vi "Day 14 Task 2 attempt 3.vi"() -> ()   [LabVIEW 2018]
uses:
  <userlib>/_OpenG.lib/array/array.llb/Remove Duplicates from 1D Array (String)__ogtk.vi
  <userlib>/_OpenG.lib/array/array.llb/Sort 1D Array (String)__ogtk.vi
  <userlib>/_OpenG.lib/array/array.llb/Reorder 2D Array2 (U64)__ogtk.vi
panel:
  out "ANSWER":u64
  out "Letter combo":string[](array[string])
  out "Letter combos it turns into":string[](array[string])
  out "Array 9":string[](array[string])
  out "Array 8":string[](array[string])
  out "Array 7":string[][](array[string])
  out "sum":u64
  out "Array 6":u64[][](array[numeric])
  out "String":string
  out "how many of each":u64[](array[numeric])
  out "step":i32
  out "Numeric":i32
  out "Array 5":u64[][](array[numeric])
  out "no. pairs":u64[](graph)
  out "Masks for 2 letter combos":i16[][](array[numeric])
  out "Array":i64[](array[numeric])
  out "2 letter combos":string[](array[string])
  out "Letters used (single)":string[](array[string])
  out "Array 4":u64[](array[numeric])
  out "Array 3":u64[](array[numeric])
  out "Polymer template":string
  out "array":string[][](array[string])
  # "3 letters = 2 pairs\nno. letters = no. pairs + 1"
  # "1749+298+161+865=3073"
  # "7 letters = 6 pairs"
  # "CB"
  # "Template:     NNCB\nAfter step 1: NCNBCHB\nAfter step 2: NBCCNBBBCBHCB\nAfter step 3: NBBBCNCCNBBNBNBBCHBHHBCHB\nAfter step 4: NBBNBNBBCCNBCNCCNBBNBBNBBBNBBNBBCBHCBHHNHCBBCBHCB"
  # "BB= BN + HB"
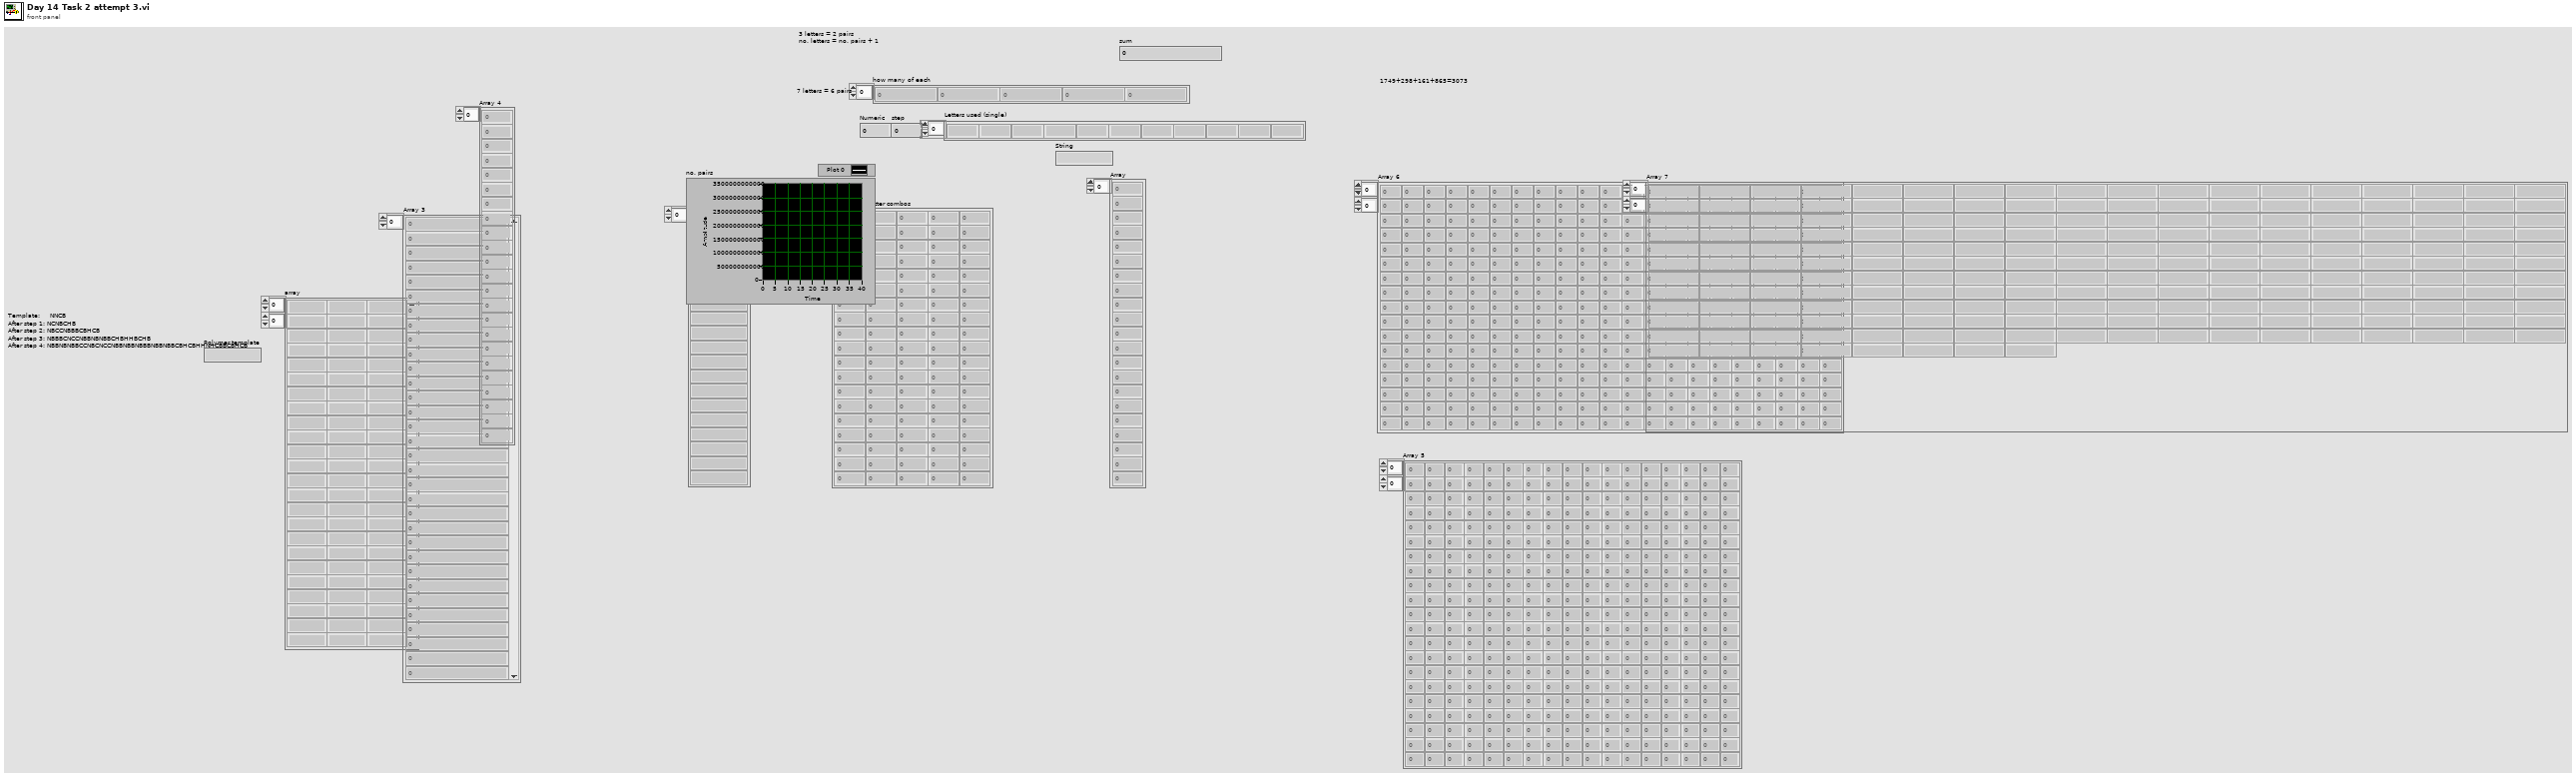
[diagram p1: front panel]
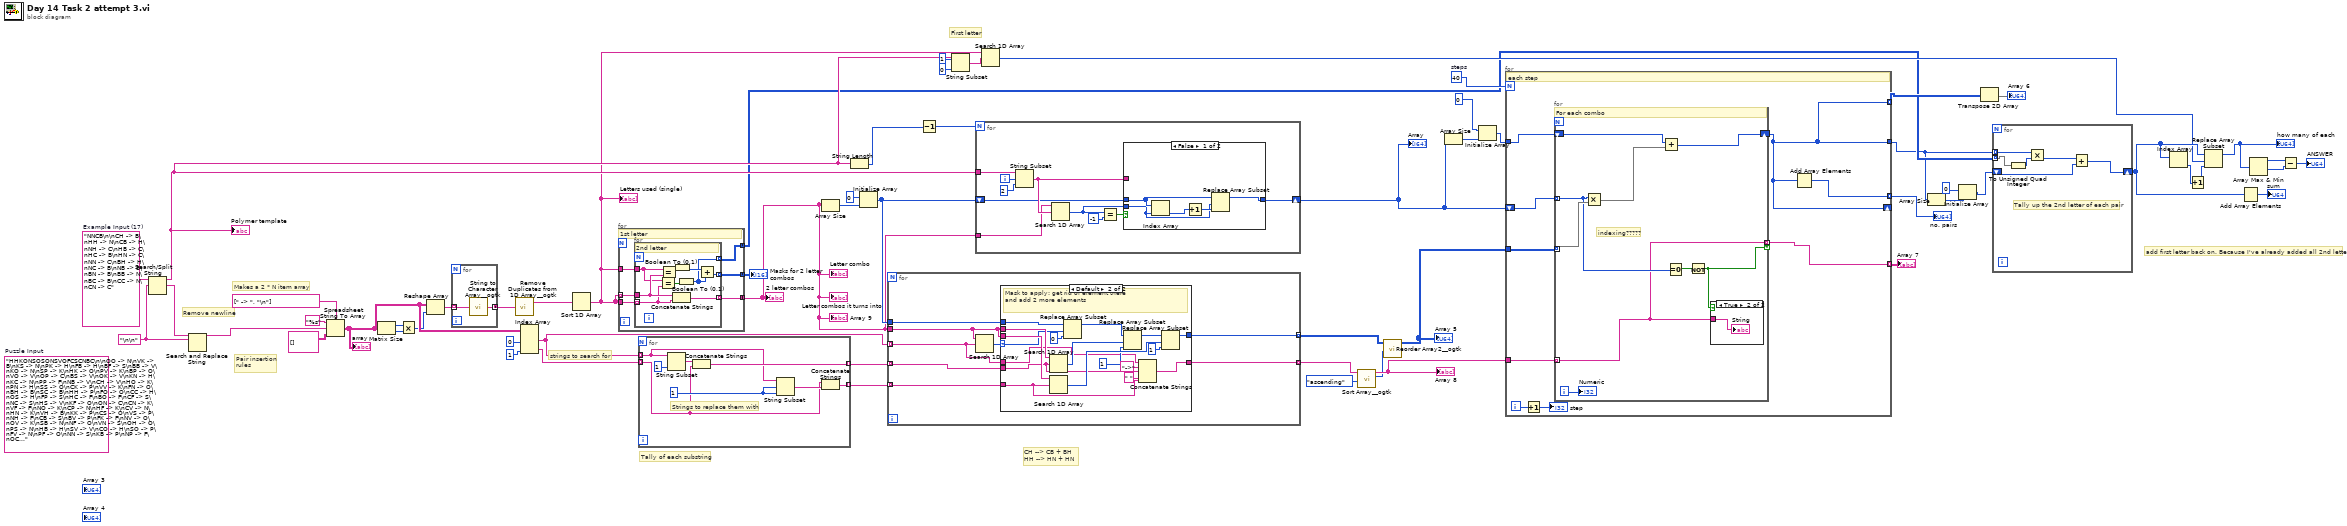
[diagram p0: block diagram]
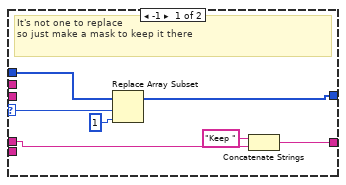
[diagram p3: hidden frame]
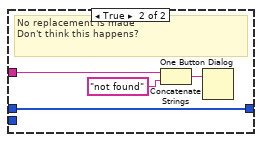
[diagram p4: hidden frame]
diagram:
  w38 = 40  # steps
  w57 = "\n\n" ("delimiter (Tab)")
  (unwired) "HHKONSOSONSVOFCSCNBC\n\nOO -> N\nVK -> B\nKS -> N\nPK -> H\nFB -> H\nBF -> S\nBB -> V\nKO -> N\nSP -> K\nHK -> O\nPV -> K\nBP -> O\nVO -> V\nOP -> C\nBS -> V\nOK -> V\nKN -> H\nKC -> N\nPP -> F\nNB -> V\nCH -> V\nHO -> K\nPN -> H\nSS -> O\nCK -> P\nVV -> K\nFN -> O\nBH -> B\nSC -> B\nHH -> P\nFO -> O\nCC -> H\nOS -> H\nFP -> S\nHC -> F\nBO -> F\nCF -> S\nNC -> S\nHS -> V\nKF -> O\nON -> C\nCN -> K\nVF -> F\nNO -> K\nCP -> N\nHF -> K\nCV -> N\nHN -> K\nVH -> B\nKK -> P\nCS -> O\nVS -> P\nNH -> F\nCB -> S\nBV -> P\nFK -> F\nNV -> O\nOV -> K\nSB -> N\nNF -> O\nVN -> S\nOH -> O\nPS -> N\nHB -> H\nSV -> V\nCO -> H\nSO -> P\nFV -> N\nPF -> O\nNN -> S\nKB -> P\nNP -> F\nOC -> S\nFS -> P\nFH -> P\nVP -> K\nBN -> O\nNS -> H\nVB -> V\nPO -> K\nKP -> N\nSN -> O\nBC -> H\nSF -> V\nPC -> O\nNK -> F\nBK -> V\nKH -> S\nSH -> S\nSK -> H\nOB -> V\nPH -> N\nPB -> C\nHV -> N\nHP -> V\nFF -> B\nOF -> P\nVC -> S\nKV -> C\nFC -> F"  # Puzzle Input
  w1 = "NNCB\n\nCH -> B\nHH -> N\nCB -> H\nNH -> C\nHB -> C\nHC -> B\nHN -> C\nNN -> C\nBH -> H\nNC -> B\nNB -> B\nBN -> B\nBB -> N\nBC -> B\nCC -> N\nCN -> C"  # Example Input (17)
  # "First letter"
  # "add first letter back on. Because I've already added all 2nd letters"
  # "strings to search for"
  # "CH --> CB + BH\nHH --> HN + HN"
  # "Pair insertion\nrules"
  # "Tally of each substring"
  # "Remove newline"
  # "Makes a 2 * N item array"
  n1 = Search/Split String(string=w1, search string/char (-)=w57) -> (substring before match=w18:string, match + rest of string=w58:string)  [unwired: 1 in, 1 out]
  "Polymer template" <- w18
  n2 = Search and Replace String(input string=w58, search string=w57) -> (result string=w56:string)  [unwired: 6 in, 3 out]
  n3 = Spreadsheet String To Array(delimiter (Tab)=string[] [" -> ", "\n"], format string="%s", spreadsheet string=w56, array type (2D Dbl)=string[][] []) -> (array=w55:string[][])
  "array" <- w55
  n4 = Matrix Size(0:w55) -> (1:w50:i32, 2:w51:i32)
  n5 = Multiply(x=w50, y=w51) -> (x*y=w49:i32)
  n6 = Reshape Array(w55, w49) -> (w47:string[])
  n7 = for {
    tunnel: w47 -> [w63] mode=indexing
    tunnel: [w62] -> w46 mode=concatenating
    n8 = call <userlib>:"String to Character Array__ogtk.vi"("Input String"=w63) -> ("Character Array"=w62:string[])
  }
  n9 = call-poly <userlib>:"Remove Duplicates from 1D Array__ogtk.vi"("Input Array"=w46) -> ("Output Array"=w27:string[])  [unwired: 1 out]
  n10 = Index Array(array=w55, index (col) #1=0 ("disabled index (col)"), index (col) #2=1 ("index (col)")) -> (element #1=w45:string[], element #2=w52:string[])  [unwired: 2 in]
  n11 = Sort 1D Array(array=w27) -> (sorted array=w15:string[])
  "Letters used (single)" <- w15
  n12 = for {
    tunnel: w15 -> [w68]
    tunnel: w15 -> [w69] mode=indexing
    tunnel: [w67] -> w39 mode=concatenating
    tunnel: w15 -> [w66]
    tunnel: [w65] -> w30 mode=concatenating
    tunnel: [w64] -> w5 mode=concatenating
    # "1st letter"
    n13 = for {
      tunnel: w69 -> [w77]
      tunnel: w68 -> [w76] mode=indexing
      tunnel: [w78] -> w67 mode=indexing
      tunnel: w66 -> [w75]
      tunnel: [w72] -> w65 mode=indexing
      tunnel: [w70] -> w64 mode=indexing
      # "2nd letter"
      n14 = Equal?(x=w75, y=w76) -> (x = y?=w74:bool[])
      n15 = Equal?(x=w75, y=w77) -> (x = y?=w73:bool[])
      n16 = Concatenate Strings(w77, w76) -> (w78:string)
      n17 = Boolean To (0,1)(Boolean=w73) -> (0, 1=w71:i16[])
      n18 = Boolean To (0,1)(Boolean=w74) -> (0, 1=w70:i16[])
      n19 = Add(x=w71, y=w70) -> (x+y=w72:i16[])
    }
  }
  "2 letter combos" <- w39
  "Masks for 2 letter combos" <- w30
  "Array 9" <- w39
  "Letter combos it turns into" <- w39
  "Letter combo" <- w39
  n20 = for {
    tunnel: w45 -> [w83] mode=indexing
    tunnel: w52 -> [w80] mode=indexing
    tunnel: [w84] -> w44 mode=indexing
    tunnel: [w79] -> w43 mode=indexing
    w82 = 1 ("length (rest)")
    # "Strings to replace them with"
    n21 = String Subset(string=w83, length (rest)=1 ("length (rest)")) -> (substring=w85:string)  [unwired: 1 in]
    n22 = Concatenate Strings(w85, w80) -> (w84:string)
    n23 = String Subset(string=w83, offset (0)=w82, length (rest)=w82) -> (substring=w81:string)
    n24 = Concatenate Strings(w80, w81) -> (w79:string)
  }
  n25 = Array Size(array=w39) -> (size(s)=w42:i32)
  n26 = String Length(string=w18) -> (length=w48:i32)
  n27 = Initialize Array(u64 0 ("element"), w42) -> (w40:u64[])
  n28 = for {
    tunnel: w39 -> [w93]
    tunnel: w45 -> [w87] mode=indexing
    tunnel: w44 -> [w92] mode=indexing
    tunnel: w43 -> [w91] mode=indexing
    tunnel: w40 -> [w90]
    tunnel: [w89] -> w23 mode=indexing
    tunnel: [w88] -> w26 mode=indexing
    n29 = Search 1D Array(1D array=w93, element=w87) -> (index of element=w94:i32)  [unwired: 1 in]
    n30 = case shown="Default" w94 {
      selector: w94 -> [w99 w116]
      tunnel: w93 -> [_ w119]
      tunnel: w93 -> [_ w118]
      tunnel: w92 -> [_ w105]
      tunnel: w91 -> [_ w103]
      tunnel: w90 -> [w101 w117]
      tunnel: [w100 w110] -> w89
      tunnel: [w96 w102] -> w88
      tunnel: w87 -> [w95 w107]
      frame -1 {
        # "It's not one to replace\nso just make a mask to keep it there"
        n31 = Replace Array Subset(array=w101, new element=i64 1 ("new element/subarray"), index=w99) -> (w100:u64[])
        n32 = Concatenate Strings("Keep " ("string"), w95) -> (w96:string)
      }
      frame Default {
        # "Mask to apply: get rid of element there\nand add 2 more elements"
        n33 = Search 1D Array(1D array=w119, element=w105) -> (index of element=w114:i32)  [unwired: 1 in]
        n34 = Search 1D Array(1D array=w118, element=w103) -> (index of element=w115:i32)  [unwired: 1 in]
        n35 = Replace Array Subset(array=w117, new element=u64 0 ("element"), index=w116) -> (w113:u64[])
        n36 = Replace Array Subset(array=w113, new element=u64 1 ("element"), index=w114) -> (w112:u64[])
        n37 = Concatenate Strings(w107, "->" ("string"), w105, " " ("string"), w103) -> (w102:string)
        n38 = Replace Array Subset(array=w112, new element=u64 1 ("element"), index=w115) -> (w110:u64[])
      }
    }
  }
  n39 = Decrement(x=w48) -> (x-1=w17:i32)
  n40 = String Subset(string=w18, offset (0)=1, length (rest)=0 ("length (rest)")) -> (substring=w16:string)
  n41 = for {
    N: w17 -> [_]
    shift-right: [w122] -> w37
    shift-left: w40 -> [w123]
    tunnel: w18 -> [w121]
    tunnel: w39 -> [w120]
    i -> [w128]
    n42 = String Subset(string=w121, offset (0)=w128, length (rest)=2 ("length (rest)")) -> (substring=w124:string)
    n43 = Search 1D Array(1D array=w120, element=w124) -> (index of element=w125:i32)  [unwired: 1 in]
    n44 = Equal?(x=w125, y=-1) -> (x = y?=w126:bool)
    n45 = case shown="False" w126 {
      tunnel: w125 -> [w130 _]
      tunnel: w124 -> [_ w137]
      tunnel: w123 -> [w133 w135]
      tunnel: [w132 w135] -> w122
      frame False {
        n46 = Index Array(array=w133, index=w130) -> (element=w134:u64)
        n47 = Increment(x=w134) -> (x+1=w131:u64)
        n48 = Replace Array Subset(array=w133, new element=w131, index=w130) -> (w132:u64[])
      }
      frame True {
        # "No replacement is made\nDon't think this happens?"
        n49 = Concatenate Strings(w137, "not found" ("string")) -> (w138:string)
        n50 = One Button Dialog(message=w138) -> ()  [unwired: 1 in, 1 out]
      }
    }
  }
  "Array" <- w37
  n51 = Search 1D Array(1D array=w15, element=w16) -> (index of element=w13:i32)  [unwired: 1 in]
  n52 = call-poly <userlib>:"Sort Array__ogtk.vi"("Order"=enum16{"ascending", "descending"}."ascending", "Array in"=w26) -> ("Sorted Pointers"=w21:i32[], "Sorted Array out"=w25:string[])  [unwired: 8 in]
  "Array 8" <- w25
  n53 = call-poly <userlib>:"Reorder Array2__ogtk.vi"("indices"=w21, "array"=w23) -> ("reordered array"=w22:u64[][])  [unwired: 9 in]
  "Array 5" <- w22
  n54 = Array Size(array=w37) -> (size(s)=w36:i32)
  n55 = Initialize Array(u64 0, w36) -> (w33:u64[])
  n56 = for {
    N: w38 -> [_]
    tunnel: w22 -> [w147]
    tunnel: [w143] -> w34 mode=indexing
    shift-right: [w140] -> _
    shift-left: w37 -> [w146]
    tunnel: w25 -> [w142]
    tunnel: w33 -> [w141]
    tunnel: [w140] -> w3
    tunnel: [w140] -> w31 mode=indexing
    tunnel: [w139] -> w28 mode=indexing
    i -> [w145]
    # "each step"
    n57 = Increment(x=w145) -> (x+1=→"step":i32)
    n58 = for {
      tunnel: w146 -> [w151] mode=indexing
      tunnel: w147 -> [w156] mode=indexing
      shift-right: [w153] -> w140
      shift-left: w141 -> [w154]
      tunnel: w142 -> [w149] mode=indexing
      tunnel: [w149] -> w139 mode=indexing if=w148
      i -> [w152]
      # "indexing?????"
      # "For each combo"
      n59 = Multiply(x=w151, y=w156) -> (x*y=w155:u64[])
      n60 = Add(x=w154, y=w155) -> (x+y=w153:u64[])
      n61 = Equal To 0?(x=w151) -> (x = 0?=w150:bool)
      n62 = Not(x=w150) -> (.not. x?=w148:bool)
      n63 = case shown="True" w148 {
        tunnel: w149 -> [_ w157]
        frame False {
        }
        frame True {
          "String" <- w157
        }
      }
      "Numeric" <- w152
    }
    n64 = Add Array Elements(numeric array=w140) -> (sum=w143:u64)
  }
  "no. pairs" <- w34
  "Array 7" <- w28
  n65 = Array Size(array=w3) -> (size(s)=w2:i32)
  n66 = Initialize Array(u64 0 ("String"), w2) -> (w4:u64[])
  n67 = Transpose 2D Array(2D array=w31) -> (transposed array=→"Array 6":u64[][])
  n68 = for {
    tunnel: w3 -> [w163] mode=indexing
    tunnel: w5 -> [w158] mode=indexing
    shift-right: [w160] -> w14
    shift-left: w4 -> [w161]
    # "Tally up the 2nd letter of each pair"
    n69 = To Unsigned Quad Integer(1:w158) -> (0:w159:u64[])
    n70 = Multiply(x=w163, y=w159) -> (x*y=w162:u64[])
    n71 = Add(x=w162, y=w161) -> (x+y=w160:u64[])
  }
  n72 = Index Array(array=w14) -> (element=w12:u64)  [unwired: 1 in]
  n73 = Increment(x=w12) -> (x+1=w11:u64)
  n74 = Replace Array Subset(array=w14, new element=w11, index=w13) -> (w10:u64[])
  "how many of each" <- w10
  n75 = Add Array Elements(numeric array=w14) -> (sum=→"sum":u64)
  n76 = Array Max & Min(array=w10) -> (max value=w20:u64, min value=w19:u64)  [unwired: 2 out]
  n77 = Subtract(x=w20, y=w19) -> (x-y=→"ANSWER":u64)
